vi "DFD Probe Check Time Response.vi"(1 "filter out":T2={"mSRate_Fs"=0.0, "mSRate_Version"="", "mSRate_Comments"="", "mSRate_OrgCoef"={"type"=enum."Undefined", "gain"=1.0, "coef a (k)"=[], "coef b (v)"=[]}, "mSRate_CurCoef"={"type"=enum."Undefined", "gain"=1.0, "coef a (k)"=[], "coef b (v)"=[]}, "mSRate_Quantized?"=FALSE, "mSRate_QCoef"={"type"=enum."Undefined", "gain"=0.0, "coef a (k)"=[], "coef b (v)"=[]}, "mSRate_QSettings"=[], "mSRate_Order"=0, "mSRate_Scaling"={"mSRate_ScaleByPowerOf2?"=FALSE, "mSRate_ScaleType"=enum."No Norm"}} {"mSRate_QSettings"."source" items=["Coef a/k"=0, "Coef b/v"=7, "Input"=1, "Output"=2, "Multiplicand"=3, "Product"=4, "Sum"=5, "Delay"=6, "Gain"=8]}) -> (0 "Boolean":bool)   [LabVIEW 2017, in "NI_DigFilterLicensed.lvlib"]
uses:
  <vilib>/addons/Digital Filter Design/NI_DigFilterLicensed.lvlib
  <vilib>/addons/Digital Filter Design/_Objects.llb/DFD Filter Obj.ctl
  <vilib>/addons/Digital Filter Design/_Objects.llb/DFD Filter Coef.ctl
  <vilib>/addons/Digital Filter Design/_Objects.llb/DFD Filter Structure Type Selector.ctl
  <vilib>/addons/Digital Filter Design/_Objects.llb/dfd_Internal Quantization Settings.ctl
  <vilib>/addons/Digital Filter Design/_Objects.llb/dfd_Internal Quantization Srcs.ctl
  <vilib>/addons/Digital Filter Design/_Objects.llb/DFD Coef Norm Type.ctl
panel:
  in  "Show Fixed-Point":bool=TRUE
  in  "Show Floating-Point":bool=TRUE
  in  "Tab Control":enum32{"Basic Info", "Impulse", "Step"}(tab)
  out "Quantized?":bool
  out "Filter Order":i32=-1
  out "Filter Structure":u16(ring) items=["Invalid Filter", "FIR Direct Form", "FIR Direct Form Transposed", "FIR Symmetric", "FIR Antisymmetric", "IIR Direct Form I", "IIR Direct Form I Transposed", "IIR Direct Form II", "IIR Direct Form II Transposed", "IIR Cascaded Second-Order Sections I", "IIR Cascaded Second-Order Sections I Transposed", "IIR Cascaded Second-Order Sections II", "IIR Cascaded Second-Order Sections II Transposed", "Lattice Allpass (basic sections)", "Lattice Allpass (one multiplier sections)", "Lattice Allpass (normalized sections)", "Lattice AR (basic sections)", "Lattice AR (one multiplier sections)", "Lattice AR (normalized sections)", "Lattice MA (minimum phase)", "Lattice MA (maximum phase)", "Lattice ARMA (basic sections)", "Lattice ARMA (one multiplier sections)", "Lattice ARMA (normalized sections)"]
  out "Impulse":T1(graph)
  out "Step":T1(graph)
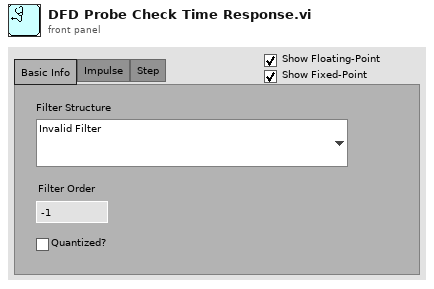
[diagram p1: front panel]
types:
  T1 = cluster{"t0":dbl, "dt":dbl, "impulse response":dbl[]}[]
  T2 = typedef "NI_DigFilterLicensed.lvlib/DFD Filter Obj.ctl" = cluster{"mSRate_Fs":dbl, "mSRate_Version":string, "mSRate_Comments":string, "mSRate_OrgCoef":T3, "mSRate_CurCoef":T3, "mSRate_Quantized?":bool, "mSRate_QCoef":T3, "mSRate_QSettings":T5[], "mSRate_Order":i32, "mSRate_Scaling":cluster{"mSRate_ScaleByPowerOf2?":bool, "mSRate_ScaleType":T7}}
  T3 = typedef "NI_DigFilterLicensed.lvlib/DFD Filter Coef.ctl" = cluster{"type":T4, "gain":dbl, "coef a (k)":dbl[], "coef b (v)":dbl[]}
  T4 = typedef "NI_DigFilterLicensed.lvlib/DFD Filter Structure Type Selector.ctl" = enum16{"Undefined", "FIR Direct Form", "FIR Direct Form Transposed", "FIR Symmetric", "FIR Antisymmetric", "IIR Direct Form I", "IIR Direct Form I Transposed", "IIR Direct Form II", "IIR Direct Form II Transposed", "IIR Cascaded Second Order Sections Form I", "IIR Cascaded Second Order Sections Form I Transposed", "IIR Cascaded Second Order Sections Form II", "IIR Cascaded Second Order Sections Form II Transposed", "Lattice Allpass (basic sections)", "Lattice Allpass (one multiplier sections)", "Lattice Allpass (normalized sections)", "Lattice AR (basic sections)", "Lattice AR (one multiplier sections)", "Lattice AR (normalized sections)", "Lattice MA (minimum phase)", "Lattice MA (maximum phase)", "Lattice ARMA (basic sections)", "Lattice ARMA (one multiplier sections)", "Lattice ARMA (normalized sections)"}
  T5 = typedef "NI_DigFilterLicensed.lvlib/dfd_Internal Quantization Settings.ctl" = cluster{"source":T6, "wl":i16, "iwl":i16, "overflow mode":enum16{"Saturation", "Wrap"}, "rounding mode":enum16{"Nearest", "Truncation"}, "signed?":bool}
  T6 = typedef "NI_DigFilterLicensed.lvlib/dfd_Internal Quantization Srcs.ctl" = u16
  T7 = typedef "NI_DigFilterLicensed.lvlib/DFD Coef Norm Type.ctl" = enum16{"No Norm", "Time Domain 1-Norm", "Time Domain 2-Norm", "Time Domain Inf-Norm"}
  T8 = cluster{"t0":dbl, "dt":dbl, "amplitudes":dbl[]}[]
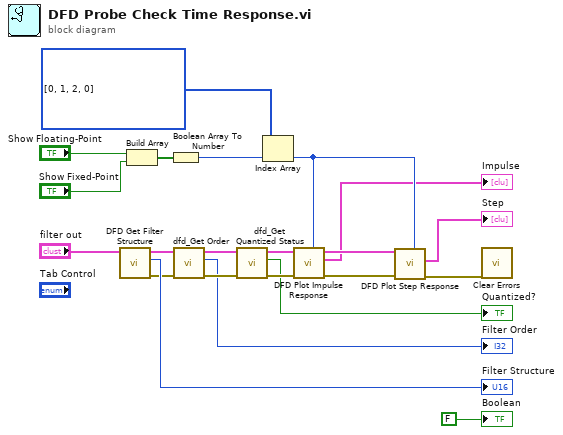
[diagram p0: block diagram]
diagram:
  w1 = u16[] [0, 1, 2, 0] items=["Auto", "Floating-point Only", "Fixed-point Only"]
  n1 = call <vilib>:"DFD Get Filter Structure.vi"("filter in"="filter out") -> ("error out"=w5:errorcluster, "structure"=→"Filter Structure":u16, "filter out"=w6:T2)  [unwired: 1 in, 7 out]
  n2 = Build Array("Show Floating-Point", "Show Fixed-Point") -> (w18:bool[])
  n3 = Boolean Array To Number(Boolean array=w18) -> (number=w17:u32)
  n4 = call <vilib>:"dfd_Get Order.vi"("error in (no error)"=w5, "filter in"=w6) -> ("error out"=w4:errorcluster, "order"=→"Filter Order":i32, "filter out"=w3:T2)  [unwired: 7 out]
  n5 = call <vilib>:"dfd_Get Quantized Status.vi"("error in (no error)"=w4, "filter in"=w3) -> ("error out"=w9:errorcluster, "quantized?"=→"Quantized?":bool, "filter out"=w10:T2)  [unwired: 7 out]
  n6 = Index Array(array=w1, index=w17) -> (element=w14:u16)
  n7 = call <vilib>:"DFD Plot Impulse Response.vi"("output option"=w14, "error in (no error)"=w9, "filter in"=w10) -> ("error out"=w21:errorcluster, "impulse response"=→"Impulse":T8, "filter out"=w22:T2)  [unwired: 2 in, 4 out]
  n8 = call <vilib>:"DFD Plot Step Response.vi"("output option"=w14, "error in (no error)"=w21, "filter in"=w22) -> ("error out"=w20:errorcluster, "step response"=→"Step":T8)  [unwired: 2 in, 5 out]
  n9 = call <vilib>:"Clear Errors.vi"("error in (no error)"=w20) -> ()  [unwired: 1 in, 6 out]
  "Boolean" <- FALSE ("Boolean")
